vi "Test Suite Filter Methods.vi"(8 "error in (no error)":errorcluster, 11 "Test Case In":refnum<class "LUnit Test Suite Tests.lvclass">) -> (0 "error out":errorcluster, 3 "Test Case Out":refnum<class "LUnit Test Suite Tests.lvclass">)   [LabVIEW 2020, in "LUnit Test Suite Tests.lvclass"]
uses:
  LUnit Test Suite Tests.lvclass
  C:/Program Files (x86)/National Instruments/LabVIEW 2020/vi.lib/Astemes/LUnit/Test Case.lvclass
  Test Case Test Double Child/Light Test Case Double.lvclass
  C:/git/astemes-lunit/source/Core/LUnit Test Case/LUnit Test Case.lvclass
  Core/Result/Type.ctl
  <vilib>/Astemes/LUnit/Test Case.lvclass/Test Case.ctl
  59ab914e-4c24-4f3b-92f7-fd9a0f9d0912.vi
  <vilib>/Astemes/LUnit/Palette/Pass.vi
  <vilib>/Astemes/LUnit/Palette/Fail.vi
  <vilib>/Astemes/LUnit/Compare Variants.vi
  <vilib>/Astemes/LUnit/Describe Comparison.vi
  <vilib>/Astemes/LUnit/Set Assertion Type.vi
  <vilib>/Astemes/LUnit/Add test result.vi
  <vilib>/Astemes/LUnit/Variant to string.vi
  <vilib>/Astemes/LUnit/LUnit Record Assertion Result.vi
  <vilib>/Astemes/LUnit/LUnit Aggregate Assertion Results.vi
  <vilib>/Astemes/LUnit/Method Result/LUnit Merge Status.vi
  <vilib>/Astemes/LUnit/LUnit Concatenate result strings.vi
  Mock Result Observer/Mock Result Observer.lvclass
  C:/git/astemes-lunit/source/Core/Result Observer/Result Observer.lvclass
  <vilib>/Utility/Data Type/Get Type Information.vi
  <vilib>/Utility/LVClass/Get LV Class Name.vi
  Core/LUnit Test Suite/LUnit Test Suite.lvclass
  Core/Result/Result.lvlib
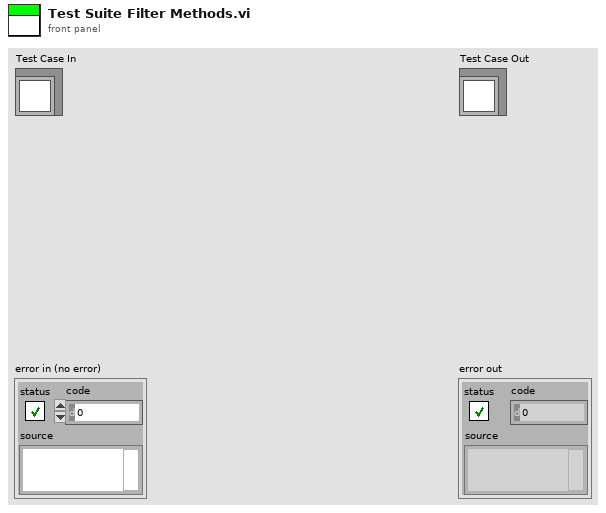
[diagram p1: front panel]
types:
  T1 = typedef "Result.lvlib/Type.ctl" = enum16{"Method", "Case", "Suite", "Pass", "Fail", "Skip", "Pass if", "Fail if", "Pass if Error", "Fail if Error", "Pass if Equal", "Fail if Equal"}
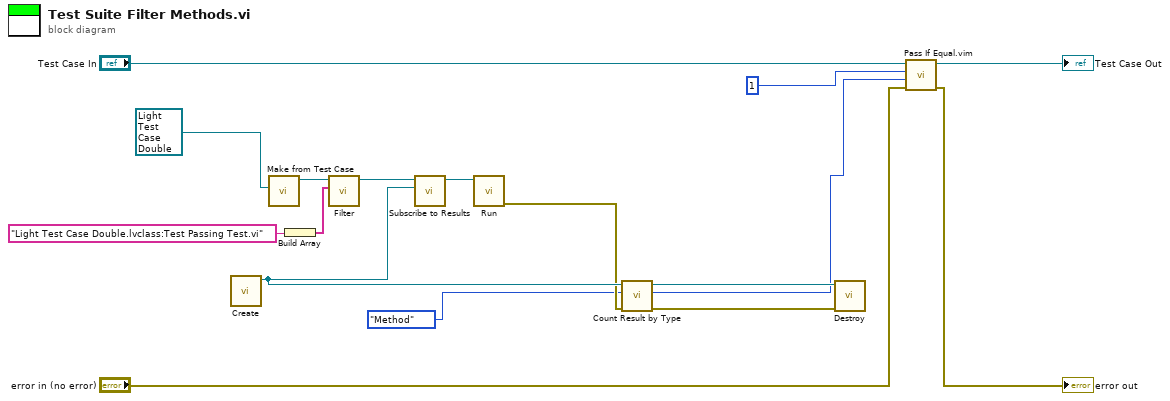
[diagram p0: block diagram]
diagram:
  n1 = call "Create.vi"() -> ("Mock Result Observer out"=w9:refnum<class "Mock Result Observer.lvclass">)  [unwired: 10 in, 1 out]
  n2 = call "Make from Test Case.vi"("LUnit Test Case"=refnum<class "Light Test Case Double.lvclass"> refnum ("Light Test Case Double.lvclass")) -> ("LUnit Test Suite Out"=w13:refnum<class "LUnit Test Suite.lvclass">)  [unwired: 9 in, 1 out]
  n3 = Build Array("Light Test Case Double.lvclass:Test Passing Test.vi" ("Methods")) -> (w5:string[])
  n4 = call-dynamic "Filter.vi"("Selected Runnables"=w5, "LUnit Test Suite In"=w13) -> ("LUnit Test Suite Out"=w10:refnum<class "LUnit Test Suite.lvclass">)  [unwired: 8 in, 1 out]
  n5 = call-dynamic "Subscribe to Results.vi"("Result Observer"=w9, "LUnit Test Suite In"=w10) -> ("LUnit Test Suite Out"=w11:refnum<class "LUnit Test Suite.lvclass">)  [unwired: 8 in, 1 out]
  n6 = call-dynamic "Run.vi"("LUnit Test Suite In"=w11) -> ("error out"=w8:errorcluster)  [unwired: 9 in, 1 out]
  n7 = call "Count Result by Type.vi"("error in (no error)"=w8, "Result Type"=Type."Method", "Mock Result Observer In"=w9) -> ("error out"=w2:errorcluster, "Numeric"=w1:i32, "Mock Result Observer Out"=w7:refnum<class "Mock Result Observer.lvclass">)  [unwired: 6 in]
  n8 = call "Destroy.vi"("error in (no error)"=w2, "Mock Result Observer in"=w7) -> ()  [unwired: 8 in, 2 out]
  n9 = call "Pass If Equal.vim"("error in (no error)"="error in (no error)", "Actual"=w1, "Expected"=1 ("Remaining Results"), "LUnit Test Case In"="Test Case In") -> ("error out"=→"error out":errorcluster, "LUnit Test Case Out"=→"Test Case Out":refnum<class "LUnit Test Suite Tests.lvclass">)  [unwired: 6 in]
